vi "GenericDriver.vi"() -> ()   [LabVIEW 2011]
panel:
  in  "stop":bool
  out "Return Value":string
  out "Bytes Read":dbl
  in  "Command":string
  out "Sent Command":string
  in  "VISA resource name":refnum<visa-resource-name>
  in  "Send Command Button":bool
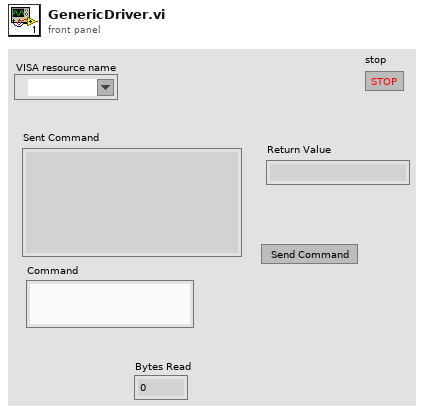
[diagram p1: front panel]
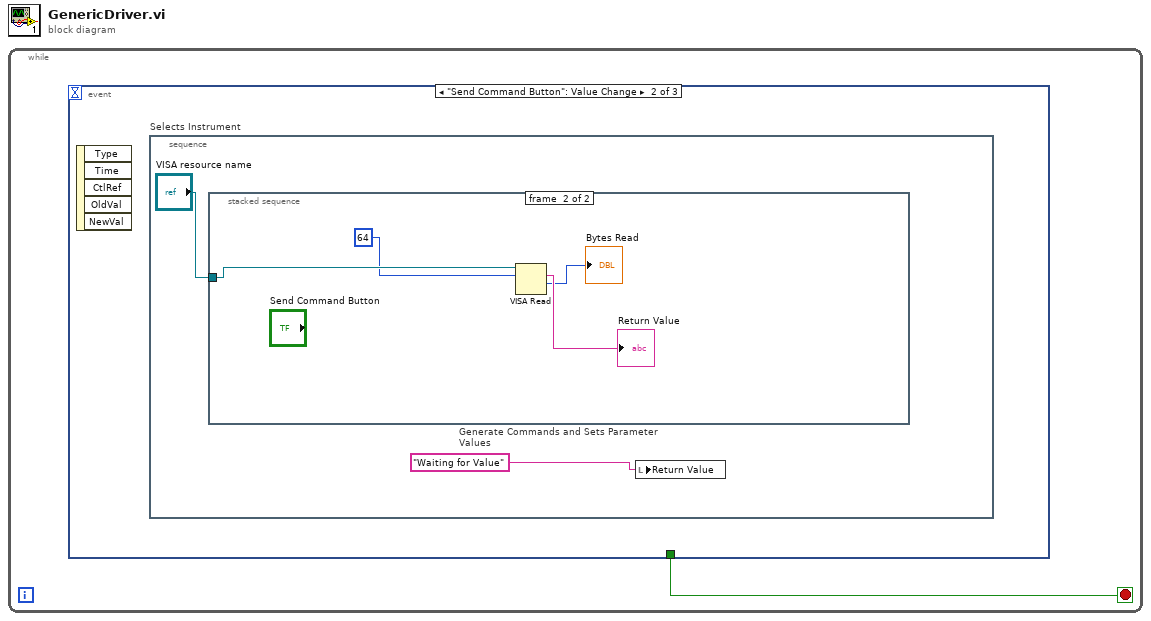
[diagram p0: block diagram]
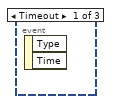
[diagram p2: hidden frame]
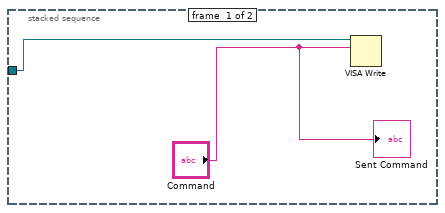
[diagram p3: hidden frame]
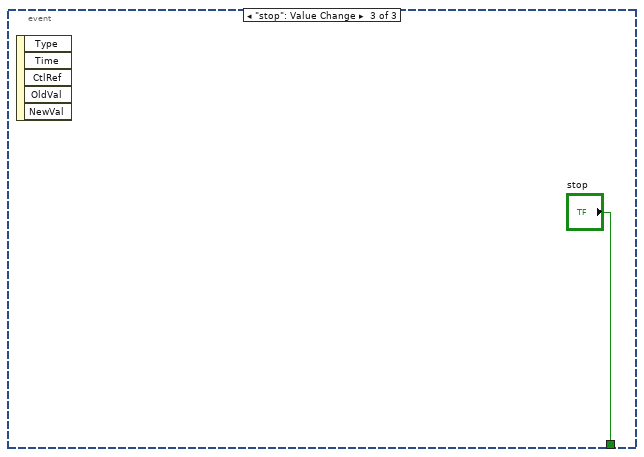
[diagram p4: hidden frame]
diagram:
  n1 = while {
    stop <- w1 stop-if-true
    n2 = event shown="[1] \"Send Command Button\": Value Change" {
      selector: _ -> [_ _ _]
      dyn-events: _ -> [_ _ _]
      timeout: _ -> [_ _ _]
      tunnel: [_ _ "stop"] -> w1
      event Timeout {
        n3 = event-data() -> ()  [unwired: 1 in, 2 out]
      }
      event "Send Command Button": Value Change {
        n4 = event-data() -> ()  [unwired: 1 in, 5 out]
        n5 = stacked-sequence "Selects Instrument" {
          frame #0 {
            n6 = stacked-sequence "Generate Commands and Sets Parameter Values" {
              tunnel: "VISA resource name" -> [w5 w9]
              frame #0 {
                n7 = VISA Write(VISA resource name=w5, write buffer="Command") -> ()  [unwired: 1 in, 3 out]
                "Sent Command" <- "Command"
              }
              frame #1 {
                n8 = VISA Read(VISA resource name=w9, byte count=64) -> (read buffer=→"Return Value":string, return count=→"Bytes Read":u32)  [unwired: 1 in, 2 out]
              }
            }
            n9 = local write "Return Value"("Waiting for Value") -> ()
          }
        }
      }
      event "stop": Value Change {
        n10 = event-data() -> ()  [unwired: 1 in, 5 out]
      }
    }
  }
